vi "Method Editor.vi"(0 "Method File:":path=path "C:/Documents and Settings/MYANG/My Documents/Ion Sniffer/Build/test.a1m") -> ()   [LabVIEW 2012]
uses:
  Type/_Run Mode.ctl
  Type/_RT Res Type.ctl
  Type/_File Type.ctl
  Type/_XML Expt.ctl
  Type/_XML Lens.ctl
  Type/_Mass Range Property.ctl
  Type/_Mass Range Parameters.ctl
  Configuration/_Global Configuration.vi
  <vilib>/Utility/config.llb/Read Key (Path).vi
  <vilib>/Utility/config.llb/Read Key (Boolean).vi
  <vilib>/Utility/config.llb/Write Key (Path).vi
  <vilib>/Utility/config.llb/Write Key (Boolean).vi
  <vilib>/Utility/config.llb/NI_LVConfig.lvlib
panel:
  in  "New":bool
  in  "Load":bool
  in  "Save":bool
  in  "Current Expt":u16(ring) items=["1"]
  in  "Tab":T1(tab)
  in  "Experiment":i32(listbox)
  in  "Insert Expt":bool
  in  "Delete Expt":bool
  in  "Import":bool
  in  "Start Time (s)":dbl=10.0 min=0.0 format="%#.3f"
  in  "# of Cycles":i32=100 min=1
  in  "Scan Type":T2=enum."Q1 Scan"
  in  "Polarity":enum32{"Positive", "Negative", "Neutral/Fast"}(radio)
  in  "Delay Time (ms)":i32 min=0
  in  "Pause Time (us)":i32=100 min=0
  out "Run Duration (min)":dbl=3.7073333333333336 format="%#.3f"
  in  "AddAllParam":bool
  in  "RemoveAllParam":bool
  in  "InsertParam":bool
  in  "ParamIdx":u16(ring) items=["Ch1 - Q1 RF", "Ch4 - Q1 DC", "Ch7 - Q1 RR", "Ch2 - Q2 RF", "Ch5 - Q2 DC", "Ch9 - Q2 RR", "Ch3 - M1 RF", "Ch20 - EV", "Ch21 - ED", "Ch10 - MO", "Ch17 - RO L1", "Ch19 - M1", "Ch18 - RO L2", "Ch22 - M2", "Ch11 - RO L3", "Ch12 - RO PF", "Ch6 - Q1", "Ch13 - CC L1", "Ch14 - CC L2", "Ch23 - CC", "Ch15 - CC L3", "Ch16 - CC L4", "Ch8 - Q2", "Ch24 - DD", "Ch32 - DISC", "Ch34 - DV", "Ch35 - DET horn", "Ch33 - HED", "Ch25 - EL", "Ch36 - LS400A", "Ch37 - LS-400A", "Ch38 - LS400B", "Ch39 - LS-400B", "Ch40 - QPS800", "Ch41 - QPS-800", "Ch26 - DG", "Ch29 - NG1", "Ch30 - HG1", "Ch28 - NG2", "Ch27 - HG2", "Ch43 - CC P", "Ch42 - SX", "Ch204 - ISV2", "Ch203 - ISV1", "Ch202 - CD", "Ch201 - CAP"]
  in  "DeleteParam":bool
  in  "User Value":dbl=3.0 format="%#.3f"
  out "DAC Value":i32=44
  in  "Parameter Table":i32(listbox)
  in  "Center/Width":bool
  out "# of Steps":i32=701
  out "Cycle Time (ms)":dbl=1202.2 format="%#.3f"
  in  "Insert MR":bool
  in  "Delete MR":bool
  out "Ramp Time (ms)":dbl=701.0 format="%#.3f"
  in  "Dwell Time (ms)":dbl=1.0 min=0.001 format="%#.3f"
  in  "Step Mass (amu)":dbl=0.5 format="%#.3f"
  in  "Stop Mass (amu)":dbl=500.0 min=0.0 format="%#.3f"
  in  "Mass Range":i32(listbox)
  in  "Start Mass (amu)":dbl=150.0 min=0.0 format="%#.3f"
  in  "MR Parameters":bool
  in  "Resolution (Q1/Q2)":T3 items=["High/High", "Medium/Medium", "Low/Low", "High/Medium", "High/Low", "Medium/High", "Medium/Low", "Low/High", "Low/Medium"]
  in  "Fixed Mass (amu)":dbl min=0.0
  # "Selected Experiment"
  # "Selected Parameter Value"
  # "Available Parameters"
  # "Selected Mass Range"
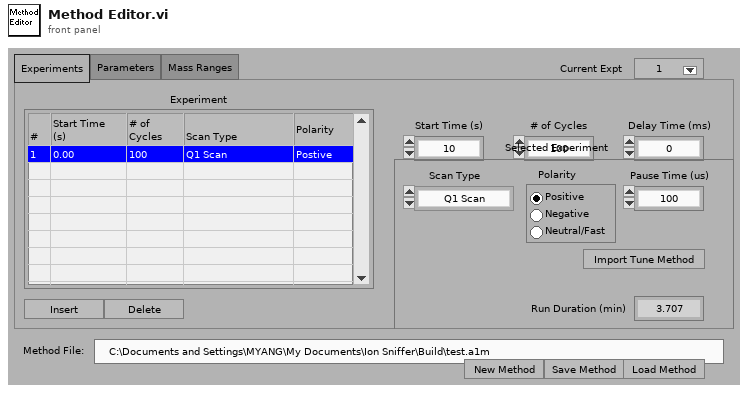
[diagram p1: front panel]
types:
  T1 = enum32{"Experiments", "Parameters", "Mass Ranges"}
  T2 = typedef "_Run Mode.ctl" = enum16{"MRM (Q1/Q2)", "Q1 Scan", "Q1 SRM", "Q2 Scan", "Q2 SRM", "Product Scan", "Precursor Scan", "Neutral Loss", "Neutral Gain"}
  T3 = typedef "_RT Res Type.ctl" = u16
  T4 = typedef "_File Type.ctl" = enum16{"Configuration", "Old Configuration", "Calibration", "Resolution", "Diagnostic Method", "Old Method", "Acq Method", "Samp List"}
  T5 = typedef "_XML Expt.ctl" = cluster{"StartT(mS)":i32, "#Cycles":i32, "PauseT(uS)":i32, "ScanType":i32, "Polarity":u8, "FixedMass":dbl, "DelayT(mS)":i32, "Active Ch":T6[], "Mass Range":T7[]}
  T6 = typedef "_XML Lens.ctl" = cluster{"Value":dbl, "ChID":u8}
  T7 = typedef "_Mass Range Property.ctl" = cluster{"Start":dbl, "Stop":dbl, "Step Size":dbl, "Steps":i32, "Dwell":dbl, "Parameters":T8[], "Res":T3}
  T8 = typedef "_Mass Range Parameters.ctl" = cluster{"Name":string, "Ch#":u8, "StartV":dbl, "StopV":dbl, "StepV":dbl, "Index":u8}
  T9 = typedef "NI_LVConfig.lvlib/Config Data RefNum.ctl" = refnum<k1>
  T10 = typedef "_RT Instrument 2.ctl" = cluster{"Table":T11[], "Instrument":string[]}
  T11 = typedef "_RT Configuration 2.ctl" = cluster{"Name":string, "Ch#":u8, "Min":dbl, "Max":dbl, "Def+":dbl, "Def-":dbl, "Offset":dbl, "Slope":dbl, "Type":u8, "Description":string, "SettleT":dbl}
  T12 = cluster{"AcqMethod":T5[], "Update":bool, "Method File:":path}
  T13 = typedef "_GUI Method.ctl" = cluster{"Lenses":T14[], "Mass Ranges":T7[], "Acquire":bool, "MCA":bool, "Q1DC EN":bool, "Q1 POL":bool, "Q3 POL":bool, "Q1 RF  EN":bool, "Averaging":bool, "Log Scale":bool, "CPS":bool, "Unit":bool, "Data Path":path, "Run Mode":T2, "Fixed Mass (amu)":dbl, "Q3DC EN":bool, "Q3 RF  EN":bool, "Negative":bool}
  T14 = typedef "_Lens Property.ctl" = cluster{"Scan Type":u8, "Scans":i32, "Time 1":dbl, "Time 2":dbl, "Value 1":dbl, "Value 2":dbl, "Step Size":dbl}
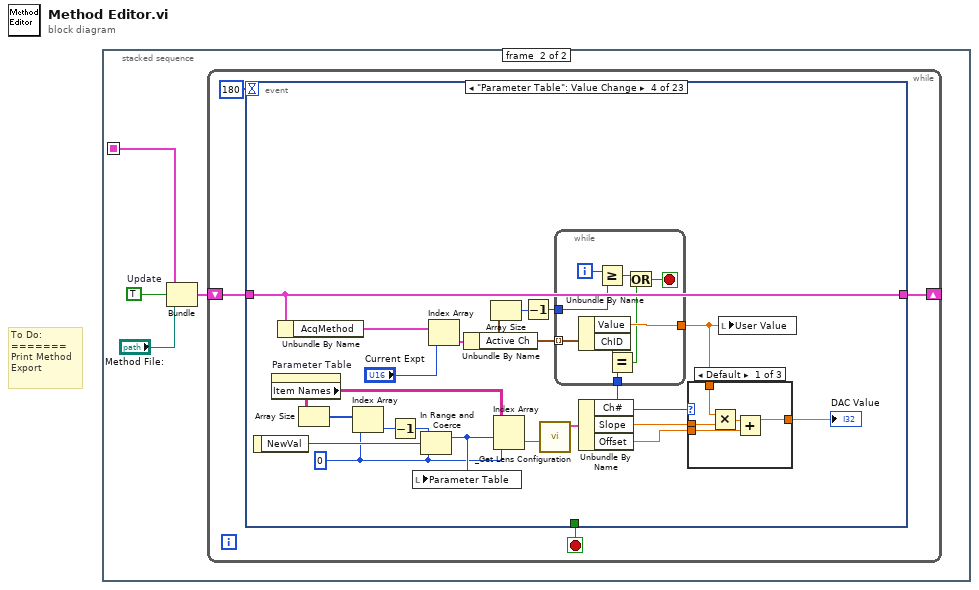
[diagram p0: block diagram]
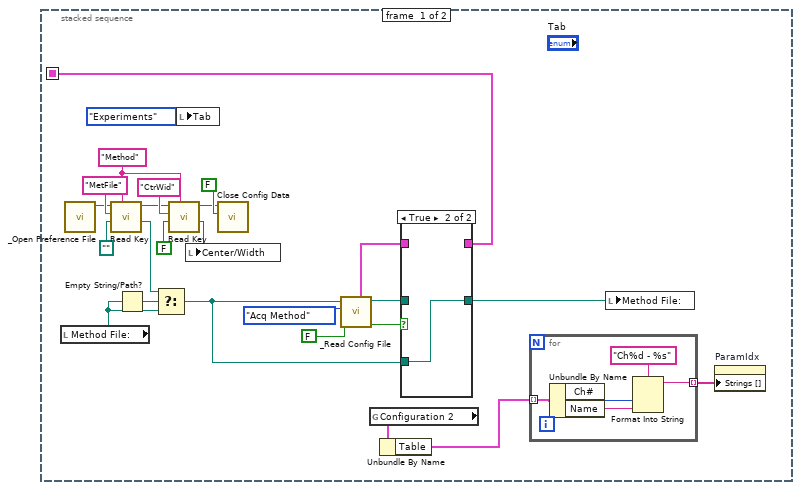
[diagram p2: hidden frame]
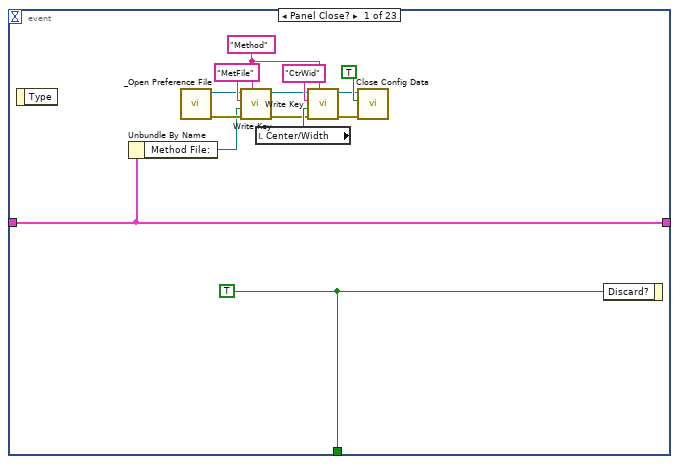
[diagram p4: hidden frame]
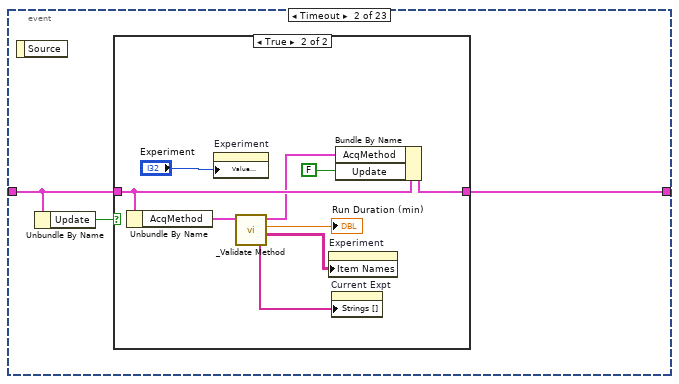
[diagram p5: hidden frame]
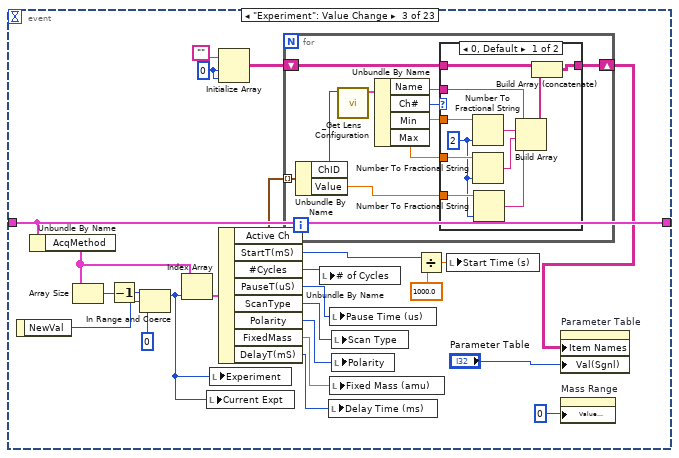
[diagram p7: hidden frame]
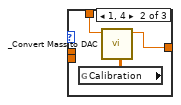
[diagram p9: hidden frame]
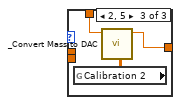
[diagram p10: hidden frame]
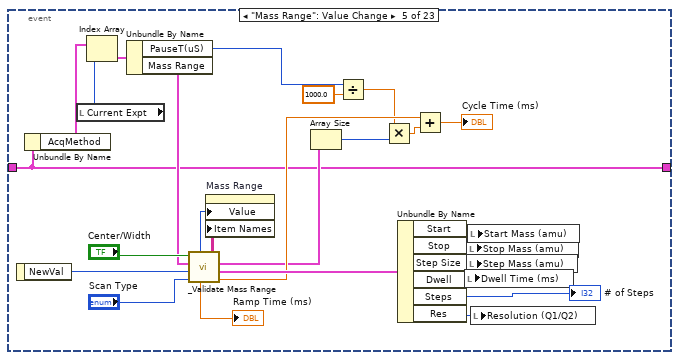
[diagram p11: hidden frame]
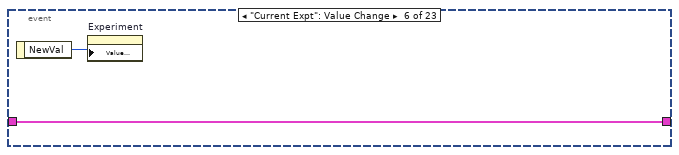
[diagram p12: hidden frame]
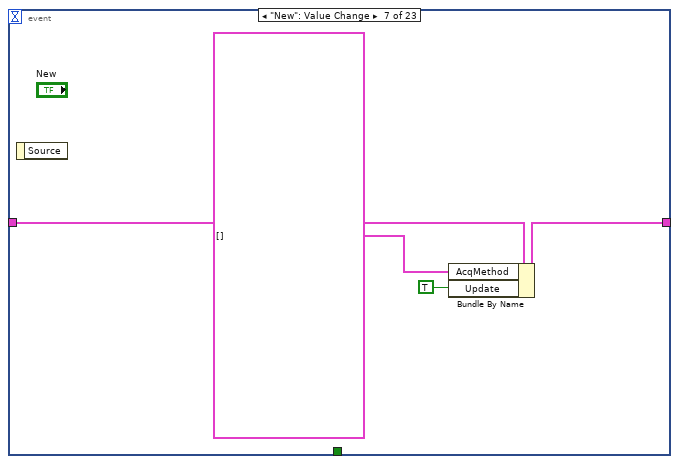
[diagram p13: hidden frame]
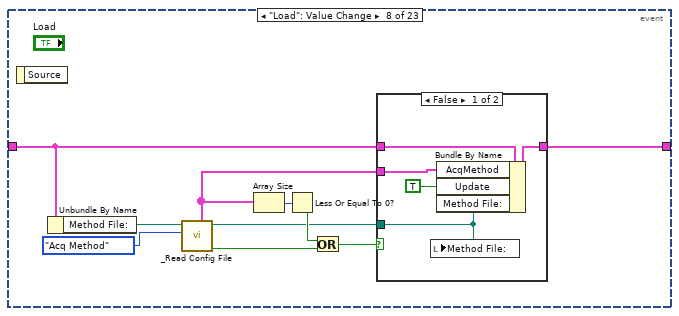
[diagram p14: hidden frame]
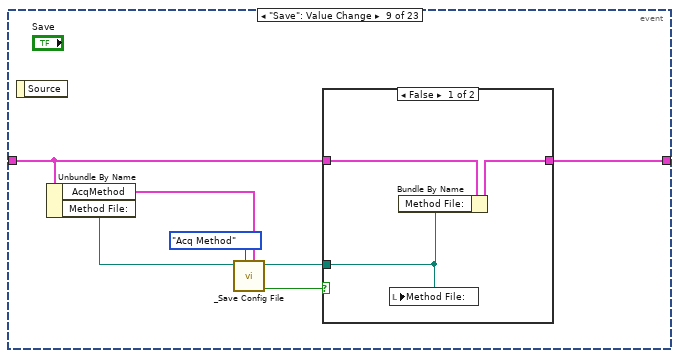
[diagram p16: hidden frame]
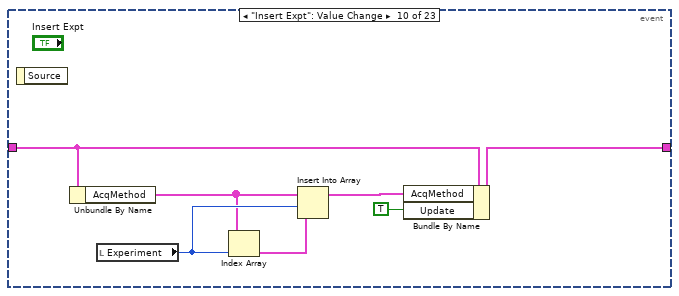
[diagram p18: hidden frame]
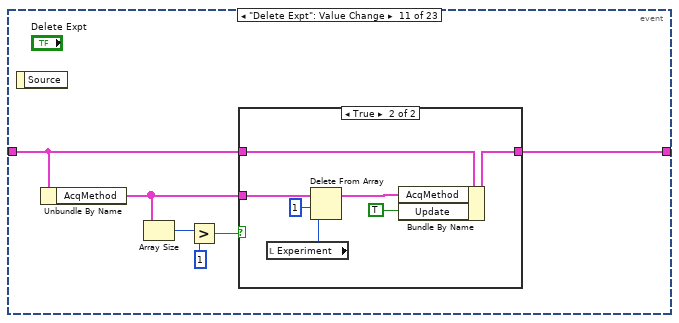
[diagram p19: hidden frame]
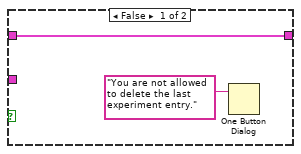
[diagram p20: hidden frame]
diagram:
  # "To Do:\n=======\nPrint Method\nExport"
  n1 = stacked-sequence {
    seq-local: [w4 _] -> [_ w34]
    frame #0 {
      w19 = "Method" ("section")
      n2 = local read "Method File:"() -> (w5:path)
      n3 = call "_Open Preference File.vi"() -> ("refnum"=w23:T9)  [unwired: 1 in, 6 out]
      n4 = call-poly <vilib>:"Read Key.vi"("section"=w19, "default value"=path "", "key"="MetFile", "refnum"=w23) -> ("value"=w11:path, "refnum out"=w14:T9)  [unwired: 1 in, 5 out]
      n5 = Empty String/Path?(string/path=w5) -> (empty?=w12:bool)
      n6 = Select(t=w11, s=w12, f=w5) -> (s? t:f=w6:path)
      n7 = call-poly <vilib>:"Read Key.vi"("section"=w19, "default value"=FALSE, "key"="CtrWid", "refnum"=w14) -> ("value"=w17:bool, "refnum out"=w13:T9)  [unwired: 1 in, 5 out]
      n8 = local write "Tab"(T1."Experiments" ("Tab")) -> ()
      n9 = local write "Center/Width"(w17) -> ()
      n10 = call <vilib>:"Close Config Data.vi"("write file if changed (T)"=FALSE ("write configuration file? (F)"), "refnum"=w13) -> ()  [unwired: 1 in, 9 out]
      n11 = call "_Read Config File.vi"("advisory dialog? (display:T)"=FALSE, "File Type (config)"=_File_Type."Acq Method", "start path  (Not A Path)"=w6) -> ("error"=w10:bool, "new file path"=w8:path, "AcqMethod"=w9:T5[])  [unwired: 6 out]
      n12 = global read "_Global Configuration.vi" "Configuration 2"() -> (w3:T10)
      n13 = Unbundle By Name(w3) -> ("Table"=w2:T11[])
      n14 = case shown="True" w10 {
        tunnel: w9 -> [w32 _]
        tunnel: [w32 _] -> w4
        tunnel: w8 -> [w31 _]
        tunnel: [w31 w33] -> w7
        tunnel: w6 -> [_ w33]
        frame False {
        }
        frame True {
        }
      }
      n15 = for {
        tunnel: w2 -> [w30] mode=indexing
        tunnel: [w26] -> w1 mode=indexing
        n16 = Unbundle By Name(w30) -> ("Ch#"=w29:u8, "Name"=w28:string)
        n17 = Format Into String(format string="Ch%d - %s", w29, w28) -> (resulting string=w26:string)  [unwired: 2 in, 1 out]
      }
      n18 = local write "Method File:"(w7) -> ()
      n19 = property on="ParamIdx" class="Ring (strict)"("Strings []"=w1) -> ()  [unwired: 2 in, 2 out]
    }
    frame #1 {
      w37 = TRUE  # Update
      n20 = Bundle("AcqMethod"=w34, "Update"=w37, "Method File:"="Method File:") -> (w36:T12)  [unwired: 1 out]
      n21 = while {
        shift-right: [w38] -> _
        shift-left: w36 -> [w40]
        stop <- w41 stop-if-true
        n22 = event shown="[3] \"Parameter Table\": Value Change" {
          selector: _ -> [_ _ _ _ _ _ _ _ _ _ _ _ _ _ _ _ _ _ _ _ _ _ _]
          dyn-events: _ -> [_ _ _ _ _ _ _ _ _ _ _ _ _ _ _ _ _ _ _ _ _ _ _]
          timeout: 180 -> [_ _ _ _ _ _ _ _ _ _ _ _ _ _ _ _ _ _ _ _ _ _ _]
          tunnel: [w55 _ _ _ _ _ _ _ _ _ _ _ _ _ _ _ _ _ _ _ _ _ _] -> w41
          tunnel: w40 -> [w50 w57 w91 w116 w156 w182 w187 w190 w205 w218 w224 w238 w294 w300 w375 w412 w434 w445 w482 w520 w529 w538 w557]
          tunnel: [w50 w58 w91 w116 w156 w182 w186 w189 w204 w216 w222 w240 w290 w299 w386 w413 w435 w446 w483 w519 w530 w537 w556] -> w38
          event Panel Close? {
            w48 = "Method" ("section")
            w55 = TRUE ("Discard?")
            n23 = event-data() -> ()  [unwired: 2 out]
            n24 = Unbundle By Name(w50) -> ("Method File:"=w49:path)
            n25 = call "_Open Preference File.vi"() -> ("error"=w51:errorcluster, "refnum"=w52:T9)  [unwired: 1 in, 5 out]
            n26 = call-poly <vilib>:"Write Key.vi"("section"=w48, "error in (no error)"=w51, "value"=w49, "key"="MetFile", "refnum"=w52) -> ("error out"=w44:errorcluster, "refnum out"=w45:T9)  [unwired: 5 out]
            n27 = local read "Center/Width"() -> (w46:bool)
            n28 = call-poly <vilib>:"Write Key.vi"("section"=w48, "error in (no error)"=w44, "value"=w46, "key"="CtrWid", "refnum"=w45) -> ("error out"=w42:errorcluster, "refnum out"=w43:T9)  [unwired: 5 out]
            n29 = call <vilib>:"Close Config Data.vi"("error in (no error)"=w42, "write file if changed (T)"=TRUE ("write configuration file? (F)"), "refnum"=w43) -> ()  [unwired: 9 out]
            n30 = event-data("Discard?"=w55) -> ()  [unwired: 1 in, 1 out]
          }
          event Timeout {
            n31 = event-data() -> ()  [unwired: 2 out]
            n32 = Unbundle By Name(w57) -> ("Update"=w56:bool)
            n33 = case shown="True" w56 {
              tunnel: w57 -> [w59 w68]
              tunnel: [w59 w66] -> w58
              frame False {
              }
              frame True {
                n34 = Unbundle By Name(w68) -> ("AcqMethod"=w65:T5[])
                n35 = property on="Experiment" class="MCListbox (strict)"("Value (Signaling)"="Experiment") -> ()  [unwired: 2 in, 2 out]
                n36 = call "_Validate Method.vi"("AcqMethod In"=w65) -> ("Expt List"=w60:string[], "Method Table"=w63:string[][], "Run Duration (min)"=→"Run Duration (min)":dbl, "AcqMethod Out"=w62:T5[])  [unwired: 3 out]
                n37 = property on="Experiment" class="MCListbox (strict)"("Item Names"=w63) -> ()  [unwired: 2 in, 2 out]
                n38 = property on="Current Expt" class="Ring (strict)"("Strings []"=w60) -> ()  [unwired: 2 in, 2 out]
                n39 = Bundle By Name(cluster=w68, "AcqMethod"=w62, "Update"=FALSE) -> (w66:T12)
              }
            }
          }
          event "Experiment": Value Change {
            w75 = 0 ("dimension size")
            n40 = event-data() -> ("NewVal"=w80:i32)  [unwired: 1 out]
            n41 = Unbundle By Name(w91) -> ("AcqMethod"=w79:T5[])
            n42 = Array Size(array=w79) -> (size(s)=w81:i32)
            n43 = Decrement(x=w81) -> (x-1=w78:i32)
            n44 = In Range and Coerce(upper limit=w78, x=w80, lower limit=0) -> (coerced(x)=w69:i32)  [unwired: 1 out]
            n45 = Index Array(array=w79, index=w69) -> (element=w92:T5)
            n46 = local write "Current Expt"(w69) -> ()
            n47 = local write "Experiment"(w69) -> ()
            n48 = Initialize Array("", w75, w75) -> (w74:string[][])
            n49 = Unbundle By Name(w92) -> ("Active Ch"=w77:T6[], "StartT(mS)"=w90:i32, "#Cycles"=w87:i32, "PauseT(uS)"=w86:i32, "ScanType"=w85:i32, "Polarity"=w84:u8, "FixedMass"=w82:dbl, "DelayT(mS)"=w83:i32)
            n50 = for {
              tunnel: w77 -> [w102] mode=indexing
              shift-right: [w98] -> w73
              shift-left: w74 -> [w99]
              n51 = Unbundle By Name(w102) -> ("ChID"=w101:u8, "Value"=w93:dbl)
              n52 = call "_Get Lens Configuration.vi"("Channel #"=w101) -> ("Lens Configuration"=w100:T11)  [unwired: 1 in, 5 out]
              n53 = Unbundle By Name(w100) -> ("Name"=w97:string, "Ch#"=w96:u8, "Min"=w95:dbl, "Max"=w94:dbl)
              n54 = case shown="0, Default" w96 {
                tunnel: w94 -> [w113 _]
                tunnel: w95 -> [w112 _]
                tunnel: [w103 w114] -> w98
                tunnel: w93 -> [w109 _]
                tunnel: w97 -> [w106 _]
                tunnel: w99 -> [w105 w114]
                frame 0, Default {
                  w108 = 2
                  n55 = Number To Fractional String(number=w112, precision (6)=w108) -> (F-format string=w107:string)  [unwired: 2 out]
                  n56 = Number To Fractional String(number=w113, precision (6)=w108) -> (F-format string=w111:string)  [unwired: 2 out]
                  n57 = Number To Fractional String(number=w109, precision (6)=w108) -> (F-format string=w110:string)  [unwired: 2 out]
                  n58 = Build Array(w106, w107, w111, w110) -> (w104:string[])
                  n59 = Build Array (concatenate)(w105, w104) -> (w103:string[][])
                }
                frame 1, 2, 4, 5, 7, 9 {
                }
              }
            }
            n60 = local write "# of Cycles"(w87) -> ()
            n61 = local write "Delay Time (ms)"(w83) -> ()
            n62 = local write "Pause Time (us)"(w86) -> ()
            n63 = local write "Fixed Mass (amu)"(w82) -> ()
            n64 = local write "Scan Type"(w85) -> ()
            n65 = local write "Polarity"(w84) -> ()
            n66 = Divide(x=w90, y=1000.0) -> (x/y=w89:dbl)
            n67 = local write "Start Time (s)"(w89) -> ()
            n68 = property on="Parameter Table" class="MCListbox (strict)"("Item Names"=w73, "Val(Sgnl)"="Parameter Table") -> ()  [unwired: 2 in, 2 out]
            n69 = property on="Mass Range" class="MCListbox (strict)"("Value (Signaling)"=0) -> ()  [unwired: 2 in, 2 out]
          }
          event "Parameter Table": Value Change {
            w125 = 0 ("lower limit")
            n70 = event-data() -> ("NewVal"=w135:i32)  [unwired: 1 out]
            n71 = property on="Parameter Table" class="MCListbox (strict)"() -> ("Item Names"=w126:string[][])  [unwired: 2 in, 2 out]
            n72 = Unbundle By Name(w116) -> ("AcqMethod"=w124:T5[])
            n73 = Array Size(array=w126) -> (size(s)=w128:i32[])
            n74 = Index Array(array=w128, index=w125) -> (element=w127:i32)
            n75 = Decrement(x=w127) -> (x-1=w134:i32)
            n76 = In Range and Coerce(upper limit=w134, x=w135, lower limit=w125) -> (coerced(x)=w129:i32)  [unwired: 1 out]
            n77 = local write "Parameter Table"(w129) -> ()
            n78 = Index Array(array=w124, index="Current Expt") -> (element=w122:T5)
            n79 = Unbundle By Name(w122) -> ("Active Ch"=w119:T6[])
            n80 = Array Size(array=w119) -> (size(s)=w118:i32)
            n81 = Index Array(array=w126, index (row)=w129, index (col)=w125) -> (element=w131:string)
            n82 = Decrement(x=w118) -> (x-1=w117:i32)
            n83 = call "_Get Lens Configuration.vi"("Name"=w131) -> ("Lens Configuration"=w130:T11)  [unwired: 1 in, 5 out]
            n84 = Unbundle By Name(w130) -> ("Ch#"=w120:u8, "Slope"=w133:dbl, "Offset"=w132:dbl)
            n85 = while {
              tunnel: w119 -> [w144] mode=indexing
              tunnel: [w143] -> w121
              tunnel: w120 -> [w141]
              tunnel: w117 -> [w139]
              i -> [w140]
              stop <- w136 stop-if-true
              n86 = Unbundle By Name(w144) -> ("Value"=w143:dbl, "ChID"=w142:u8)
              n87 = Greater Or Equal?(x=w140, y=w139) -> (x >= y?=w138:bool)
              n88 = Equal?(x=w142, y=w141) -> (x = y?=w137:bool)
              n89 = Or(x=w138, y=w137) -> (x .or. y?=w136:bool)
            }
            n90 = case shown="Default" w120 {
              tunnel: w121 -> [w148 w151 w154]
              tunnel: [w145 w150 w153] -> w115
              tunnel: w133 -> [w147 _ _]
              tunnel: w132 -> [w146 _ _]
              frame Default {
                n91 = Multiply(x=w148, y=w147) -> (x*y=w149:dbl)
                n92 = Add(x=w149, y=w146) -> (x+y=w145:dbl)
              }
              frame 1, 4 {
                n93 = global read "_Global Configuration.vi" "Calibration"() -> (w152:dbl[][])
                n94 = call "_Convert Mass to DAC.vi"("Calibration Table"=w152, "Mass"=w151) -> ("DAC Value"=w150:dbl)  [unwired: 2 in, 3 out]
              }
              frame 2, 5 {
                n95 = global read "_Global Configuration.vi" "Calibration 2"() -> (w155:dbl[][])
                n96 = call "_Convert Mass to DAC.vi"("Calibration Table"=w155, "Mass"=w154) -> ("DAC Value"=w153:dbl)  [unwired: 2 in, 3 out]
              }
            }
            "DAC Value" <- w115
            n97 = local write "User Value"(w121) -> ()
          }
          event "Mass Range": Value Change {
            n98 = event-data() -> ("NewVal"=w175:i32)  [unwired: 1 out]
            n99 = Unbundle By Name(w156) -> ("AcqMethod"=w163:T5[])
            n100 = local read "Current Expt"() -> (w162:u16)
            n101 = Index Array(array=w163, index=w162) -> (element=w181:T5)
            n102 = Unbundle By Name(w181) -> ("PauseT(uS)"=w159:i32, "Mass Range"=w160:T7[])
            n103 = call "_Validate Mass Range.vi"("Run Mode"="Scan Type", "Ranges #"=w175, "Mass Ranges"=w160, "Center/Width"="Center/Width") -> ("Cycle Time (ms)"=w165:dbl, "Current Mass Range"=w174:T7, "Mass Ranges Out"=w158:T7[], "Table out"=w171:string[][], "Ramp Time (ms)"=→"Ramp Time (ms)":dbl, "Ranges # Out"=w172:i32)
            n104 = property on="Mass Range" class="MCListbox (strict)"("Value"=w172, "Item Names"=w171) -> ()  [unwired: 2 in, 2 out]
            n105 = Array Size(array=w158) -> (size(s)=w167:i32)
            n106 = Divide(x=w159, y=1000.0) -> (x/y=w157:dbl)
            n107 = Multiply(x=w157, y=w167) -> (x*y=w166:dbl)
            n108 = Unbundle By Name(w174) -> ("Start"=w179:dbl, "Stop"=w180:dbl, "Step Size"=w176:dbl, "Dwell"=w178:dbl, "Steps"=→"# of Steps":i32, "Res"=w169:T3)
            n109 = Add(x=w165, y=w166) -> (x+y=→"Cycle Time (ms)":dbl)
            n110 = local write "Dwell Time (ms)"(w178) -> ()
            n111 = local write "Stop Mass (amu)"(w180) -> ()
            n112 = local write "Step Mass (amu)"(w176) -> ()
            n113 = local write "Start Mass (amu)"(w179) -> ()
            n114 = local write "Resolution (Q1/Q2)"(w169) -> ()
          }
          event "Current Expt": Value Change {
            n115 = event-data() -> ("NewVal"=w183:u16)  [unwired: 1 out]
            n116 = property on="Experiment" class="MCListbox (strict)"("Value (Signaling)"=w183) -> ()  [unwired: 2 in, 2 out]
          }
          event "New": Value Change {
            n117 = event-data() -> ()  [unwired: 2 out]
            n118 = Bundle By Name(cluster=w187, "AcqMethod"=T5[] [], "Update"=TRUE) -> (w186:T12)
          }
          event "Load": Value Change {
            n119 = event-data() -> ()  [unwired: 2 out]
            n120 = Unbundle By Name(w190) -> ("Method File:"=w197:path)
            n121 = call "_Read Config File.vi"("File Type (config)"=_File_Type."Acq Method", "start path  (Not A Path)"=w197) -> ("error"=w193:bool, "new file path"=w192:path, "AcqMethod"=w188:T5[])  [unwired: 1 in, 6 out]
            n122 = Array Size(array=w188) -> (size(s)=w195:i32)
            n123 = Less Or Equal To 0?(x=w195) -> (x <= 0?=w194:bool)
            n124 = Or(x=w194, y=w193) -> (x .or. y?=w191:bool)
            n125 = case shown="False" w191 {
              tunnel: w192 -> [w198 _]
              tunnel: w190 -> [w202 w203]
              tunnel: [w201 w203] -> w189
              tunnel: w188 -> [w200 _]
              frame False {
                n126 = local write "Method File:"(w198) -> ()
                n127 = Bundle By Name(cluster=w202, "AcqMethod"=w200, "Update"=TRUE, "Method File:"=w198) -> (w201:T12)
              }
              frame True {
              }
            }
          }
          event "Save": Value Change {
            n128 = event-data() -> ()  [unwired: 2 out]
            n129 = Unbundle By Name(w205) -> ("AcqMethod"=w208:T5[], "Method File:"=w209:path)
            n130 = call "_Save Config File.vi"("AcqMethod"=w208, "File Type (config)"=_File_Type."Acq Method", "start path  (Not A Path)"=w209) -> ("error"=w207:bool, "new file path"=w206:path)  [unwired: 5 in, 2 out]
            n131 = case shown="False" w207 {
              tunnel: w206 -> [w211 _]
              tunnel: w205 -> [w213 w214]
              tunnel: [w212 w214] -> w204
              frame False {
                n132 = local write "Method File:"(w211) -> ()
                n133 = Bundle By Name(cluster=w213, "Method File:"=w211) -> (w212:T12)
              }
              frame True {
              }
            }
          }
          event "Insert Expt": Value Change {
            n134 = event-data() -> ()  [unwired: 2 out]
            n135 = Unbundle By Name(w218) -> ("AcqMethod"=w219:T5[])
            n136 = local read "Experiment"() -> (w221:i32)
            n137 = Index Array(array=w219, index=w221) -> (element=w220:T5)
            n138 = Insert Into Array(array=w219, index=w221, new element=w220) -> (w217:T5[])
            n139 = Bundle By Name(cluster=w218, "AcqMethod"=w217, "Update"=TRUE) -> (w216:T12)
          }
          event "Delete Expt": Value Change {
            n140 = event-data() -> ()  [unwired: 2 out]
            n141 = Unbundle By Name(w224) -> ("AcqMethod"=w223:T5[])
            n142 = Array Size(array=w223) -> (size(s)=w226:i32)
            n143 = Greater?(x=w226, y=1) -> (0:w225:bool)
            n144 = case shown="True" w225 {
              tunnel: w224 -> [w228 w233]
              tunnel: w223 -> [_ w235]
              tunnel: [w228 w231] -> w222
              frame False {
                n145 = One Button Dialog(message="You are not allowed to delete the last experiment entry.") -> ()  [unwired: 2 out]
              }
              frame True {
                n146 = local read "Experiment"() -> (w234:i32)
                n147 = Delete From Array(array=w235, length=1, index=w234) -> (array with subset deleted=w232:T5[])  [unwired: 1 out]
                n148 = Bundle By Name(cluster=w233, "AcqMethod"=w232, "Update"=TRUE) -> (w231:T12)
              }
            }
          }
          event "Import": Value Change {
            n149 = event-data() -> ()  [unwired: 2 out]
            n150 = Unbundle By Name(w238) -> ("AcqMethod"=w237:T5[], "Method File:"=w247:path)
            n151 = call "_Read Config File.vi"("File Type (config)"=_File_Type."Diagnostic Method", "start path  (Not A Path)"=w247) -> ("error"=w243:bool, "GUI Method"=w239:T13)  [unwired: 1 in, 7 out]
            n152 = Unbundle By Name(w239) -> ("Lenses"=w241:T14[])
            n153 = Array Size(array=w241) -> (size(s)=w245:i32)
            n154 = Less Or Equal To 0?(x=w245) -> (x <= 0?=w244:bool)
            n155 = Or(x=w244, y=w243) -> (x .or. y?=w242:bool)
            n156 = case shown="False" w242 {
              tunnel: w238 -> [w272 w279]
              tunnel: [w271 w279] -> w240
              tunnel: w239 -> [w269 _]
              tunnel: w237 -> [w255 _]
              frame False {
                n157 = global read "_Global Configuration.vi" "Configuration 2"() -> (w251:T10)
                n158 = local read "Current Expt"() -> (w254:u16)
                n159 = Unbundle By Name(w269) -> ("Lenses"=w250:T14[], "Mass Ranges"=w260:T7[], "Run Mode"=w259:T2, "Fixed Mass (amu)"=w258:dbl, "Negative"=w257:bool)
                n160 = Unbundle By Name(w251) -> ("Table"=w249:T11[])
                n161 = Index Array(array=w255, index=w254) -> (element=w266:T5)
                n162 = Index Array(array=w250, index=0) -> (element=w268:T14)
                n163 = Unbundle By Name(w268) -> ("Scans"=w265:i32, "Time 1"=w264:dbl, "Time 2"=w263:dbl)
                n164 = for {
                  tunnel: w250 -> [w278] mode=indexing
                  tunnel: w249 -> [w277] mode=indexing
                  tunnel: [w273] -> w248 mode=indexing
                  n165 = Unbundle By Name(w278) -> ("Value 1"=w276:dbl)
                  n166 = Unbundle By Name(w277) -> ("Ch#"=w274:u8)
                  n167 = Bundle By Name(cluster=T6 {"Value"=0.0, "ChID"=0} ("Lens"), "ChID"=w274, "Value"=w276) -> (w273:T6)
                }
                n168 = Boolean To (0,1)(Boolean=w257) -> (0, 1=w256:i16)
                n169 = Multiply(x=w263, y=1000.0) -> (x*y=w261:dbl)
                n170 = Bundle By Name(cluster=w266, "Active Ch"=w248, "#Cycles"=w265, "DelayT(mS)"=w264, "PauseT(uS)"=w261, "Mass Range"=w260, "ScanType"=w259, "FixedMass"=w258, "Polarity"=w256) -> (w253:T5)
                n171 = Replace Array Subset(array=w255, new element=w253, index=w254) -> (w252:T5[])
                n172 = Bundle By Name(cluster=w272, "AcqMethod"=w252, "Update"=TRUE) -> (w271:T12)
              }
              frame True {
              }
            }
          }
          event "# of Cycles", "Pause Time (us)", "Delay Time (ms)", "Start Time (s)", "Polarity", "Fixed Mass (amu)": Value Change {
            n173 = event-data() -> ()  [unwired: 2 out]
            n174 = local read "Current Expt"() -> (w289:u16)
            n175 = Unbundle By Name(w294) -> ("AcqMethod"=w293:T5[])
            n176 = Index Array(array=w293, index=w289) -> (element=w295:T5)
            n177 = Multiply(x=1000.0, y="Start Time (s)") -> (x*y=w283:dbl)
            n178 = Bundle By Name(cluster=w295, "#Cycles"="# of Cycles", "PauseT(uS)"="Pause Time (us)", "DelayT(mS)"="Delay Time (ms)", "StartT(mS)"=w283, "Polarity"="Polarity", "FixedMass"="Fixed Mass (amu)") -> (w292:T5)
            n179 = Replace Array Subset(array=w293, new element=w292, index=w289) -> (w291:T5[])
            n180 = Bundle By Name(cluster=w294, "AcqMethod"=w291, "Update"=TRUE) -> (w290:T12)
          }
          event "Center/Width": Value Change {
            n181 = local read "Center/Width"() -> (w308:bool)
            n182 = event-data() -> ()  [unwired: 2 out]
            n183 = local read "Scan Type"() -> (w297:T2)
            n184 = local read "Current Expt"() -> (w302:u16)
            n185 = Unbundle By Name(w300) -> ("AcqMethod"=w304:T5[])
            n186 = case shown="\"Product Scan\", Default" w297 {
              selector: w297 -> [_ w331 _ _ _]
              tunnel: [_ w329 _ _ _] -> w314
              tunnel: [w315 w335 string[] ["\n#", "Q1\n(amu)", "Q2\n(amu)", "Dwell\n(ms)", "", "", "Res"] ("Column Header Strings[]") string[] ["\n#", "Q1\n(amu)", "Ignored", "Dwell\n(ms)", "", "", "Res"] ("Column Header Strings[]") string[] ["\n#", "Ignored", "Q2\n(amu)", "Dwell\n(ms)", "", "", "Res"] ("Column Header Strings[]")] -> w313
              tunnel: ["Step Mass (amu)" "Step Mass (amu)" "Not Used" "Not Used" "Not Used"] -> w312
              tunnel: [w316 w333 "Q2 Mass (amu)" "Not Used" "Q2 Mass (amu)"] -> w311
              tunnel: [w317 w332 "Q1 Mass (amu)" "Q1 Mass (amu)" "Not Used"] -> w310
              tunnel: ["Fixed Mass (amu)" w330 "Fixed Mass (amu)" "Fixed Mass (amu)" "Fixed Mass (amu)"] -> w309
              tunnel: w308 -> [w318 w328 _ _ _]
              tunnel: [w319 w329 w345 _ TRUE] -> w307
              tunnel: [w319 w329 w345 TRUE _] -> w306
              tunnel: [w319 w329 _ _ _] -> w305
              frame "Q1 Scan", "Q2 Scan" {
                w319 = TRUE
                n187 = case shown="False" w318 {
                  tunnel: [string[] ["\n#", "Center\n(amu)", "Width\n(amu)", "Step\n(amu)", "Dwell\n(ms)", "# of\nSteps", "Res"] ("Column Header Strings[]") string[] ["\n#", "Start\n(amu)", "Stop\n(amu)", "Step\n(amu)", "Dwell\n(ms)", "# of\nSteps", "Res"] ("Column Header Strings[]")] -> w315
                  tunnel: ["Width (amu)" "Stop Mass (amu)"] -> w316
                  tunnel: ["Center Mass (amu)" "Start Mass (amu)"] -> w317
                  frame True {
                  }
                  frame False {
                  }
                }
              }
              frame "Product Scan", Default {
                w329 = TRUE
                n188 = case shown="True" w328 {
                  tunnel: [string[] ["\n#", "Center\n(amu)", "Width\n(amu)", "Step\n(amu)", "Dwell\n(ms)", "# of\nSteps", "Res"] ("Column Header Strings[]") string[] ["\n#", "Start\n(amu)", "Stop\n(amu)", "Step\n(amu)", "Dwell\n(ms)", "# of\nSteps", "Res"] ("Column Header Strings[]")] -> w335
                  tunnel: ["Width (amu)" "Stop Mass (amu)"] -> w333
                  tunnel: ["Center Mass (amu)" "Start Mass (amu)"] -> w332
                  frame True {
                  }
                  frame False {
                  }
                }
                n189 = case shown="\"Precursor Scan\"" w331 {
                  tunnel: ["Precursor Mass (amu)" "Neutral Mass (amu)" "Daughter Mass (amu)"] -> w330
                  frame "Product Scan" {
                  }
                  frame Default {
                  }
                  frame "Precursor Scan" {
                  }
                }
              }
              frame "MRM (Q1/Q2)" {
                w345 = TRUE
              }
              frame "Q1 SRM" {
              }
              frame "Q2 SRM" {
              }
            }
            n190 = Index Array(array=w304, index=w302) -> (element=w298:T5)
            n191 = Bundle By Name(cluster=w298, "ScanType"=w297) -> (w296:T5)
            n192 = Replace Array Subset(array=w304, new element=w296, index=w302) -> (w303:T5[])
            n193 = Bundle By Name(cluster=w300, "AcqMethod"=w303, "Update"=TRUE) -> (w299:T12)
            n194 = property on="Fixed Mass (amu)" class="DigNum (strict)"("Visible"=w314, "Caption.Text"=w309) -> ()  [unwired: 2 in, 2 out]
            n195 = property on="Mass Range" class="MCListbox (strict)"("ColHdrString"=w313) -> ()  [unwired: 2 in, 2 out]
            n196 = property on="Start Mass (amu)" class="DigNum (strict)"("Caption.Text"=w310, "Visible"=w306) -> ()  [unwired: 2 in, 2 out]
            n197 = property on="Stop Mass (amu)" class="DigNum (strict)"("Caption.Text"=w311, "Visible"=w307) -> ()  [unwired: 2 in, 2 out]
            n198 = property on="Step Mass (amu)" class="DigNum (strict)"("Caption.Text"=w312, "Visible"=w305) -> ()  [unwired: 2 in, 2 out]
            n199 = property on="Center/Width" class="Bool (strict)"("Visible"=w305) -> ()  [unwired: 2 in, 2 out]
          }
          event "User Value": Value Change {
            n200 = event-data() -> ()  [unwired: 2 out]
            n201 = local read "Parameter Table"() -> (w382:i32)
            n202 = Unbundle By Name(w375) -> ("AcqMethod"=w366:T5[])
            n203 = property on="Parameter Table" class="MCListbox (strict)"() -> ("Item Names"=w381:string[][])  [unwired: 2 in, 2 out]
            n204 = local read "Current Expt"() -> (w363:u16)
            n205 = Index Array(array=w366, index=w363) -> (element=w368:T5)
            n206 = Index Array(array=w381, index (row)=w382, index (col)=0 ("disabled index (col)")) -> (element=w385:string)
            n207 = call "_Get Lens Configuration.vi"("Name"=w385) -> ("Lens Configuration"=w384:T11)  [unwired: 1 in, 5 out]
            n208 = Unbundle By Name(w368) -> ("Active Ch"=w373:T6[])
            n209 = Array Size(array=w373) -> (size(s)=w377:i32)
            n210 = Unbundle By Name(w384) -> ("Min"=w379:dbl, "Max"=w378:dbl, "Ch#"=w374:u8)
            n211 = Decrement(x=w377) -> (x-1=w376:i32)
            n212 = while {
              tunnel: w373 -> [w387] mode=indexing
              tunnel: w374 -> [w393]
              tunnel: w376 -> [w392]
              tunnel: [w388] -> w372
              tunnel: [w387] -> w371
              i -> [w388]
              stop <- w389 stop-if-true
              n213 = Unbundle By Name(w387) -> ("ChID"=w394:u8)
              n214 = Greater Or Equal?(x=w388, y=w392) -> (x >= y?=w391:bool)
              n215 = Equal?(x=w394, y=w393) -> (x = y?=w390:bool)
              n216 = Or(x=w391, y=w390) -> (x .or. y?=w389:bool)
            }
            n217 = In Range and Coerce(upper limit=w378, x="User Value", lower limit=w379) -> (coerced(x)=w370:dbl)  [unwired: 1 out]
            n218 = local write "User Value"(w370) -> ()
            n219 = Bundle By Name(cluster=w371, "Value"=w370) -> (w369:T6)
            n220 = Replace Array Subset(array=w373, new element=w369, index=w372) -> (w367:T6[])
            n221 = Bundle By Name(cluster=w368, "Active Ch"=w367) -> (w365:T5)
            n222 = property on="Experiment" class="MCListbox (strict)"("Value (Signaling)"=w363) -> ()  [unwired: 2 in, 2 out]
            n223 = Replace Array Subset(array=w366, new element=w365, index=w363) -> (w364:T5[])
            n224 = Bundle By Name(cluster=w375, "AcqMethod"=w364) -> (w386:T12)
          }
          event "DeleteParam": Value Change {
            n225 = event-data() -> ()  [unwired: 2 out]
            n226 = local read "Parameter Table"() -> (w400:i32)
            n227 = Unbundle By Name(w412) -> ("AcqMethod"=w410:T5[])
            n228 = property on="Parameter Table" class="MCListbox (strict)"() -> ("Item Names"=w399:string[][])  [unwired: 2 in, 2 out]
            n229 = local read "Current Expt"() -> (w405:u16)
            n230 = Index Array(array=w410, index=w405) -> (element=w411:T5)
            n231 = Index Array(array=w399, index (row)=w400, index (col)=0 ("disabled index (col)")) -> (element=w403:string)
            n232 = Unbundle By Name(w411) -> ("Active Ch"=w396:T6[])
            n233 = call "_Get Lens Configuration.vi"("Name"=w403) -> ("Lens Configuration"=w402:T11)  [unwired: 1 in, 5 out]
            n234 = Array Size(array=w396) -> (size(s)=w397:i32)
            n235 = Unbundle By Name(w402) -> ("Ch#"=w404:u8)
            n236 = Greater Than 0?(x=w397) -> (x > 0?=w407:bool)
            n237 = Decrement(x=w397) -> (x-1=w398:i32)
            n238 = while {
              tunnel: w396 -> [w416] mode=indexing
              tunnel: w398 -> [w420]
              tunnel: w404 -> [w415]
              tunnel: [w414] -> w395
              i -> [w414]
              stop <- w417 stop-if-true
              n239 = Unbundle By Name(w416) -> ("ChID"=w421:u8)
              n240 = Greater Or Equal?(x=w414, y=w420) -> (x >= y?=w419:bool)
              n241 = Equal?(x=w421, y=w415) -> (x = y?=w418:bool)
              n242 = Or(x=w419, y=w418) -> (x .or. y?=w417:bool)
            }
            n243 = case shown="True" w407 {
              tunnel: w396 -> [w422 w426]
              tunnel: [w422 w425] -> w406
              tunnel: w405 -> [_ w424]
              tunnel: w395 -> [_ w423]
              frame False {
              }
              frame True {
                n244 = property on="Experiment" class="MCListbox (strict)"("Value (Signaling)"=w424) -> ()  [unwired: 2 in, 2 out]
                n245 = Delete From Array(array=w426, length=1, index=w423) -> (array with subset deleted=w425:T6[])  [unwired: 1 out]
              }
            }
            n246 = Bundle By Name(cluster=w411, "Active Ch"=w406) -> (w409:T5)
            n247 = Replace Array Subset(array=w410, new element=w409, index=w405) -> (w408:T5[])
            n248 = Bundle By Name(cluster=w412, "AcqMethod"=w408) -> (w413:T12)
          }
          event "RemoveAllParam": Value Change {
            n249 = event-data() -> ()  [unwired: 2 out]
            n250 = Unbundle By Name(w434) -> ("AcqMethod"=w432:T5[])
            n251 = local read "Current Expt"() -> (w428:u16)
            n252 = Index Array(array=w432, index=w428) -> (element=w433:T5)
            n253 = property on="Experiment" class="MCListbox (strict)"("Value (Signaling)"=w428) -> ()  [unwired: 2 in, 2 out]
            n254 = Bundle By Name(cluster=w433, "Active Ch"=T6[] []) -> (w431:T5)
            n255 = Replace Array Subset(array=w432, new element=w431, index=w428) -> (w430:T5[])
            n256 = Bundle By Name(cluster=w434, "AcqMethod"=w430) -> (w435:T12)
          }
          event "AddAllParam": Value Change {
            n257 = event-data() -> ()  [unwired: 2 out]
            n258 = Unbundle By Name(w445) -> ("AcqMethod"=w444:T5[])
            n259 = local read "Current Expt"() -> (w441:u16)
            n260 = Index Array(array=w444, index=w441) -> (element=w440:T5)
            n261 = global read "_Global Configuration.vi" "Configuration 2"() -> (w439:T10)
            n262 = Unbundle By Name(w440) -> ("Polarity"=w437:u8)
            n263 = Unbundle By Name(w439) -> ("Table"=w438:T11[])
            n264 = property on="Experiment" class="MCListbox (strict)"("Value (Signaling)"=w441) -> ()  [unwired: 2 in, 2 out]
            n265 = for {
              tunnel: w437 -> [w452]
              tunnel: w438 -> [w451] mode=indexing
              tunnel: [w448] -> w436 mode=indexing
              n266 = Unbundle By Name(w451) -> ("Ch#"=w450:u8)
              n267 = case shown="1" w452 {
                tunnel: w451 -> [w454 w456]
                tunnel: [w453 w455] -> w449
                frame 0, Default {
                  n268 = Unbundle By Name(w454) -> ("Def+"=w453:dbl)
                }
                frame 1 {
                  n269 = Unbundle By Name(w456) -> ("Def-"=w455:dbl)
                }
              }
              n270 = Bundle By Name(cluster=T6 {"Value"=0.0, "ChID"=0} ("Lens"), "ChID"=w450, "Value"=w449) -> (w448:T6)
            }
            n271 = Bundle By Name(cluster=w440, "Active Ch"=w436) -> (w443:T5)
            n272 = Replace Array Subset(array=w444, new element=w443, index=w441) -> (w442:T5[])
            n273 = Bundle By Name(cluster=w445, "AcqMethod"=w442) -> (w446:T12)
          }
          event "InsertParam": Value Change {
            n274 = event-data() -> ()  [unwired: 2 out]
            n275 = Unbundle By Name(w482) -> ("AcqMethod"=w481:T5[])
            n276 = local read "Parameter Table"() -> (w462:i32)
            n277 = property on="Parameter Table" class="MCListbox (strict)"() -> ("Item Names"=w461:string[][])  [unwired: 2 in, 2 out]
            n278 = local read "Current Expt"() -> (w471:u16)
            n279 = global read "_Global Configuration.vi" "Configuration 2"() -> (w478:T10)
            n280 = Unbundle By Name(w478) -> ("Table"=w477:T11[])
            n281 = Index Array(array=w481, index=w471) -> (element=w469:T5)
            n282 = Index Array(array=w461, index (row)=w462, index (col)=0 ("disabled index (col)")) -> (element=w465:string)
            n283 = Unbundle By Name(w469) -> ("Polarity"=w470:u8, "Active Ch"=w459:T6[])
            n284 = call "_Get Lens Configuration.vi"("Name"=w465) -> ("Lens Configuration"=w464:T11)  [unwired: 1 in, 5 out]
            n285 = Index Array(array=w477, index="ParamIdx") -> (element=w475:T11)
            n286 = property on="Experiment" class="MCListbox (strict)"("Value (Signaling)"=w471) -> ()  [unwired: 2 in, 2 out]
            n287 = Unbundle By Name(w464) -> ("Ch#"=w466:u8)
            n288 = Array Size(array=w459) -> (size(s)=w458:i32)
            n289 = Unbundle By Name(w475) -> ("Ch#"=w473:u8)
            n290 = Decrement(x=w458) -> (x-1=w460:i32)
            n291 = case shown="1" w470 {
              tunnel: w475 -> [w493 w495]
              tunnel: [w492 w494] -> w472
              frame 0, Default {
                n292 = Unbundle By Name(w493) -> ("Def+"=w492:dbl)
              }
              frame 1 {
                n293 = Unbundle By Name(w495) -> ("Def-"=w494:dbl)
              }
            }
            n294 = while {
              tunnel: w459 -> [w486] mode=indexing
              tunnel: w460 -> [w490]
              tunnel: w466 -> [w485]
              tunnel: [w484] -> w457
              i -> [w484]
              stop <- w487 stop-if-true
              n295 = Unbundle By Name(w486) -> ("ChID"=w491:u8)
              n296 = Greater Or Equal?(x=w484, y=w490) -> (x >= y?=w489:bool)
              n297 = Equal?(x=w491, y=w485) -> (x = y?=w488:bool)
              n298 = Or(x=w489, y=w488) -> (x .or. y?=w487:bool)
            }
            n299 = Bundle By Name(cluster=T6 {"Value"=0.0, "ChID"=0} ("Lens"), "ChID"=w473, "Value"=w472) -> (w468:T6)
            n300 = Insert Into Array(array=w459, index=w457, new element=w468) -> (w467:T6[])
            n301 = Bundle By Name(cluster=w469, "Active Ch"=w467) -> (w480:T5)
            n302 = Replace Array Subset(array=w481, new element=w480, index=w471) -> (w479:T5[])
            n303 = Bundle By Name(cluster=w482, "AcqMethod"=w479) -> (w483:T12)
          }
          event "Start Mass (amu)", "Stop Mass (amu)", "Dwell Time (ms)", "Step Mass (amu)": Value Change {
            n304 = event-data() -> ()  [unwired: 2 out]
            n305 = Unbundle By Name(w520) -> ("AcqMethod"=w500:T5[])
            n306 = local read "Current Expt"() -> (w499:u16)
            n307 = local read "Center/Width"() -> (w505:bool)
            n308 = Index Array(array=w500, index=w499) -> (element=w502:T5)
            n309 = local read "Scan Type"() -> (w506:T2)
            n310 = Unbundle By Name(w502) -> ("Mass Range"=w503:T7[])
            n311 = Index Array(array=w503, index="Mass Range") -> (element=w517:T7)
            n312 = Unbundle By Name(w517) -> ("Step Size"=w515:dbl)
            n313 = Not Equal?(x="Step Mass (amu)", y=w515) -> (x != y?=w508:bool)
            n314 = call "_Convert Center Width.vi"("Center/Width"=w505, "Run Mode"=w506, "StepMass Changed"=w508, "Step Mass"="Step Mass (amu)", "Stop Mass"="Stop Mass (amu)", "Start Mass"="Start Mass (amu)") -> ("Step Mass (amu)"=w511:dbl, "Stop Mass (amu)"=w510:dbl, "Start Mass (amu)"=w509:dbl)  [unwired: 1 out]
            n315 = Bundle By Name(cluster=w517, "Dwell"="Dwell Time (ms)", "Start"=w509, "Stop"=w510, "Step Size"=w511, "Res"="Resolution (Q1/Q2)") -> (w516:T7)
            n316 = Replace Array Subset(array=w503, new element=w516, index="Mass Range") -> (w501:T7[])
            n317 = Bundle By Name(cluster=w502, "Mass Range"=w501) -> (w498:T5)
            n318 = Replace Array Subset(array=w500, new element=w498, index=w499) -> (w497:T5[])
            n319 = Bundle By Name(cluster=w520, "AcqMethod"=w497, "Update"=TRUE) -> (w519:T12)
          }
          event "Insert MR": Value Change {
            n320 = event-data() -> ()  [unwired: 2 out]
            n321 = Unbundle By Name(w529) -> ("AcqMethod"=w524:T5[])
            n322 = local read "Current Expt"() -> (w523:u16)
            n323 = Index Array(array=w524, index=w523) -> (element=w526:T5)
            n324 = local read "Mass Range"() -> (w532:i32)
            n325 = Unbundle By Name(w526) -> ("Mass Range"=w528:T7[])
            n326 = Index Array(array=w528, index=w532) -> (element=w531:T7)
            n327 = Insert Into Array(array=w528, index=w532, new element=w531) -> (w525:T7[])
            n328 = Bundle By Name(cluster=w526, "Mass Range"=w525) -> (w527:T5)
            n329 = Replace Array Subset(array=w524, new element=w527, index=w523) -> (w522:T5[])
            n330 = Bundle By Name(cluster=w529, "AcqMethod"=w522, "Update"=TRUE) -> (w530:T12)
          }
          event "Delete MR": Value Change {
            n331 = event-data() -> ()  [unwired: 2 out]
            n332 = Unbundle By Name(w538) -> ("AcqMethod"=w533:T5[])
            n333 = local read "Current Expt"() -> (w534:u16)
            n334 = Index Array(array=w533, index=w534) -> (element=w535:T5)
            n335 = Unbundle By Name(w535) -> ("Mass Range"=w536:T7[])
            n336 = Array Size(array=w536) -> (size(s)=w540:i32)
            n337 = Greater?(x=w540, y=1) -> (0:w539:bool)
            n338 = case shown="True" w539 {
              tunnel: w538 -> [w542 w552]
              tunnel: w536 -> [_ w554]
              tunnel: [w542 w551] -> w537
              tunnel: w535 -> [_ w549]
              tunnel: w534 -> [_ w547]
              tunnel: w533 -> [_ w546]
              frame False {
                n339 = One Button Dialog(message="You are not allowed to delete the last mass range entry.") -> ()  [unwired: 2 out]
              }
              frame True {
                n340 = local read "Mass Range"() -> (w553:i32)
                n341 = Delete From Array(array=w554, length=1, index=w553) -> (array with subset deleted=w548:T7[])  [unwired: 1 out]
                n342 = Bundle By Name(cluster=w549, "Mass Range"=w548) -> (w550:T5)
                n343 = Replace Array Subset(array=w546, new element=w550, index=w547) -> (w545:T5[])
                n344 = Bundle By Name(cluster=w552, "Update"=TRUE, "AcqMethod"=w545) -> (w551:T12)
              }
            }
          }
          event "MR Parameters": Value Change {
            n345 = event-data() -> ()  [unwired: 2 out]
            n346 = Unbundle By Name(w557) -> ("AcqMethod"=w559:T5[])
            n347 = local read "Current Expt"() -> (w558:u16)
            n348 = Index Array(array=w559, index=w558) -> (element=w560:T5)
            n349 = Unbundle By Name(w560) -> ("Mass Range"=w565:T7[])
            n350 = local read "Mass Range"() -> (w566:i32)
            n351 = call "Mass Dependent Parameters.vi"("Current Mass Range"=w566, "Mass Ranges"=w565) -> ("Mass Ranges Out"=w561:T7[])  [unwired: 5 out]
            n352 = Bundle By Name(cluster=w560, "Mass Range"=w561) -> (w564:T5)
            n353 = Replace Array Subset(array=w559, new element=w564, index=w558) -> (w563:T5[])
            n354 = Bundle By Name(cluster=w557, "Update"=TRUE, "AcqMethod"=w563) -> (w556:T12)
          }
        }
      }
    }
  }
